vi "Read Failed Count.vi"(11 "Method Result In":refnum<class "Method Result.lvclass">) -> (2 "Failed count":i32, 3 "Method Result Out":refnum<class "Method Result.lvclass">)   [LabVIEW 2020, in "Method Result.lvclass"]
uses:
  Method Result.lvclass
  Assertion Result/Public/TypeDefs/Status.ctl
  Assertion Result/Assertion Result.lvclass
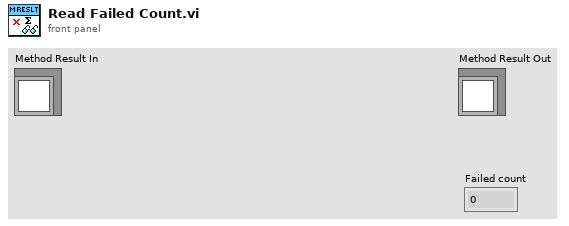
[diagram p1: front panel]
types:
  T1 = typedef "Assertion Result.lvclass/Status.ctl" = enum16{"Pass", "Fail", "Error", "Skipped", "Setup Error", "Broken", "Teardown Error"}
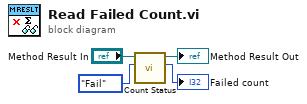
[diagram p0: block diagram]
diagram:
  n1 = call "Count Status.vi"("Status"=Status."Fail", "Method Result in"="Method Result In") -> ("Count"=→"Failed count":i32, "Method Result out"=→"Method Result Out":refnum<class "Method Result.lvclass">)  [unwired: 8 in]
